vi "Milan Box.vi"   [LabVIEW 2019]
uses:
  <vilib>/httpClient/POSTBuffer.vi
  <vilib>/httpClient/LabVIEWHTTPClient.lvlib
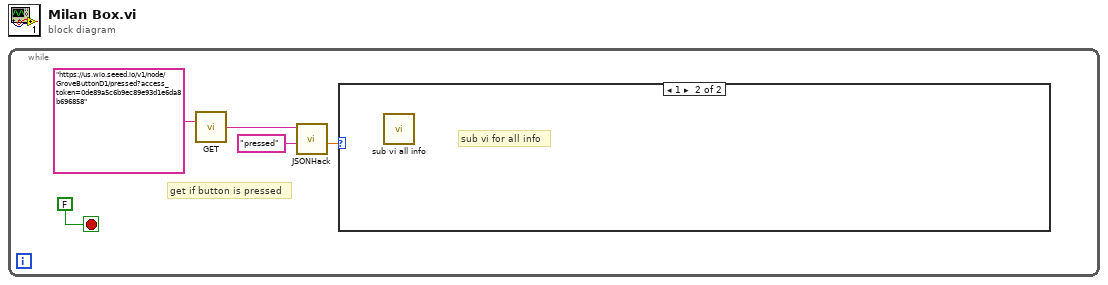
[diagram p0: block diagram]
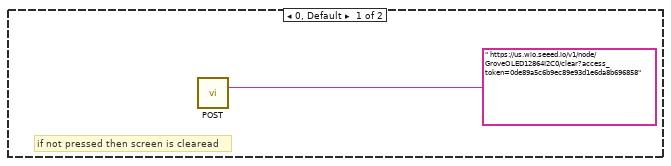
[diagram p2: hidden frame]
diagram:
  n1 = while {
    stop <- FALSE stop-if-true
    # "get if button is pressed"
    n2 = call <vilib>:"GET.vi"("url"="https://us.wio.seeed.io/v1/node/GroveButtonD1/pressed?access_token=0de89a5c6b9ec89e93d1e6da8b696858") -> ("body"=w4:string)  [unwired: 11 in, 3 out]
    n3 = call "JSONHack.vi"("search name"="pressed", "JSON in"=w4) -> ("Property (num)"=w3:dbl)  [unwired: 6 in, 3 out]
    n4 = case shown="1" w3 {
      frame 0, Default {
        # "if not pressed then screen is clearead"
        n5 = call-poly <vilib>:"POST.vi"("url"=" https://us.wio.seeed.io/v1/node/GroveOLED12864I2C0/clear?access_token=0de89a5c6b9ec89e93d1e6da8b696858") -> ()  [unwired: 11 in, 4 out]
      }
      frame 1 {
        # "sub vi for all info"
        n6 = call "sub vi all info.vi"() -> ()  [unwired: 12 in]
      }
    }
  }
